vi "VIRef_Find Global Point of Control.vi"(8 "Error":errorcluster, 9 "Control Position":T2, 10 "Control Name":string, 11 "VI":refnum<vi>) -> (0 "Error Out":errorcluster, 2 "Found Out":bool, 3 "Global Point Out":T3, 5 "Global Position Out":T1)   [LabVIEW 2020]
uses:
  TypeDefs_Utility/Cluster_Pos_Top Left position.ctl
  TypeDefs_Utility/ENUM RB_Pos_Quadrant Position.ctl
  <vilib>/Utility/miscctls.llb/LVRectTypeDef.ctl
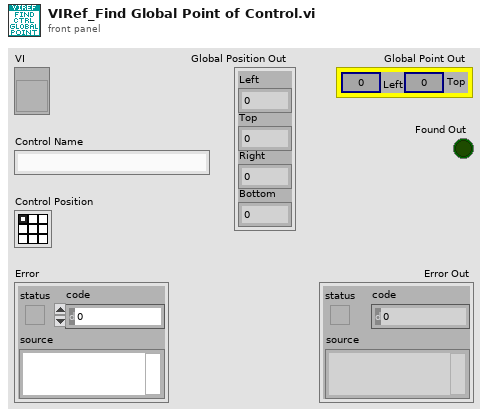
[diagram p1: front panel]
types:
  T1 = typedef "LVRectTypeDef.ctl" = cluster{"Left":i16, "Top":i16, "Right":i16, "Bottom":i16}
  T2 = typedef "ENUM RB_Pos_Quadrant Position.ctl" = enum32{"LFT-TOP", "MID-TOP", "RGT-TOP", "LFT-CTR", "MID-CTR", "RGT-CTR", "LFT-BOT", "MID-BOT", "RGT-BOT"}
  T3 = typedef "Cluster_Pos_Top Left position.ctl" = cluster{"Left":i16, "Top":i16}
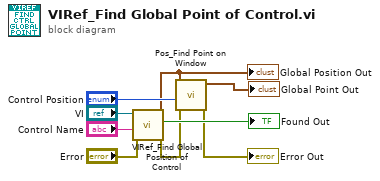
[diagram p0: block diagram]
diagram:
  n1 = call "VIRef_Find Global Position of Control.vi"("Error"="Error", "Control Name"="Control Name", "VI"="VI") -> ("Error Out"=w2:errorcluster, "Found Out"=→"Found Out":bool, "Global Position Out"=w8:T1)  [unwired: 6 in]
  "Global Position Out" <- w8
  n2 = call "Pos_Find Point on Window.vi"("Error"=w2, "Position"="Control Position", "Window"=w8) -> ("Error Out"=→"Error Out":errorcluster, "Point Out"=→"Global Point Out":T3)  [unwired: 7 in]
